vi "Write All.vi"(8 "Error In":errorcluster, 10 "Data":u8[](array[numeric]), 11 "SFTP File In":refnum<class "SFTP File.lvclass">) -> (0 "Error Out":errorcluster, 2 "Block Write Count":i64, 3 "SFTP File Out":refnum<class "SFTP File.lvclass">)   [LabVIEW 2018, in "Toolkit.lvlib" / "SFTP File.lvclass"]
doc: "Writes all of the bytes to a remote SFTP file in a series of smaller 30KB chunks, or blocks."
uses:
  SFTP File.lvclass
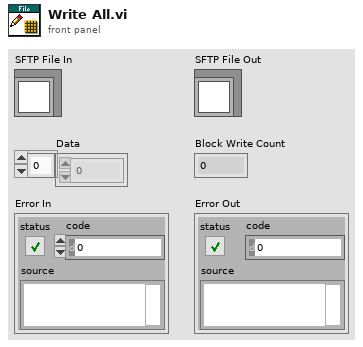
[diagram p1: front panel]
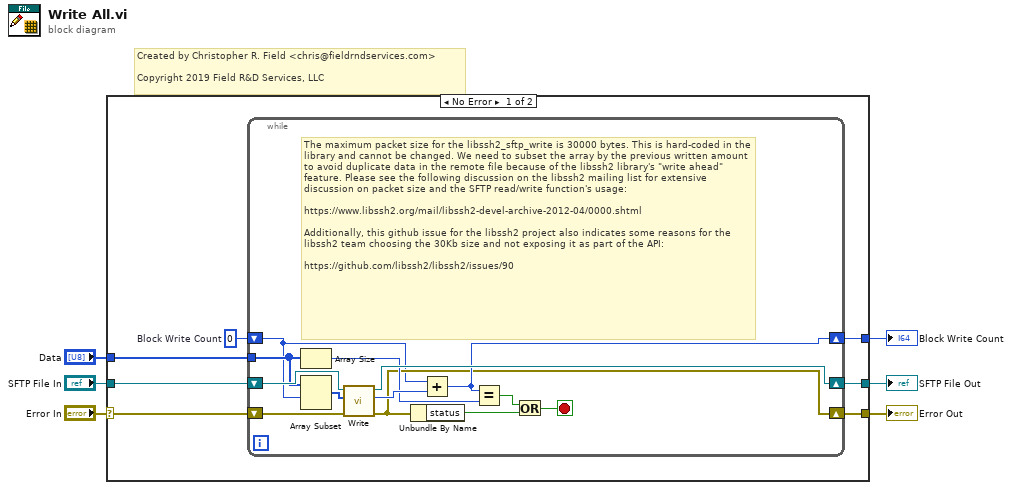
[diagram p0: block diagram]
diagram:
  # "Created by Christopher R. Field <chris@fieldrndservices.com>\n\nCopyright 2019 Field R&D Services, LLC"
  n1 = case shown="No Error" "Error In" {
    selector: "Error In" -> [w7 w27]
    tunnel: "Data" -> [w12 _]
    tunnel: "SFTP File In" -> [w11 w28]
    tunnel: [w10 _] -> w4
    tunnel: [w9 w28] -> w3
    tunnel: [w8 w27] -> w2
    frame No Error {
      w13 = i64 0  # Block Write Count
      n2 = while {
        tunnel: w12 -> [w20]
        shift-right: [w24] -> w9
        shift-left: w11 -> [w26]
        shift-right: [w16] -> w8
        shift-left: w7 -> [w25]
        shift-right: [w22] -> w10
        shift-left: w13 -> [w14]
        stop <- w17 stop-if-true
        # "The maximum packet size for the libssh2_sftp_write is 30000 bytes. This is hard-coded in the library and cannot be changed. We need to subset the array by the previous written amount to avoid duplicate data in the remote file because of the libssh2 library's \"write ahead\" feature. Please see the following discussion on the libssh2 mailing list for extensive discussion on packet size and the SFTP read/write function's usage:\n\nhttps://www.libssh2.org/mail/libssh2-devel-archive-2012-04/0000.shtml\n\nAdditionally, this github issue for the libssh2 project also indicates some reasons for the libssh2 team choosing the 30Kb size and not exposing it as part of the API:\n\nhttps://github.com/libssh2/libssh2/issues/90"
        n3 = Array Size(array=w20) -> (size(s)=w21:i32)
        n4 = Array Subset(array=w20, index=w14) -> (w19:u8[])  [unwired: 1 in]
        n5 = call "Write.vi"("Error In"=w25, "Data"=w19, "SFTP File In"=w26) -> ("Error Out"=w16:errorcluster, "Count"=w23:i64, "SFTP File Out"=w24:refnum<class "SFTP File.lvclass">)  [unwired: 6 in]
        n6 = Unbundle By Name(w16) -> ("status"=w15:bool)
        n7 = Add(x=w14, y=w23) -> (x+y=w22:i64)
        n8 = Equal?(x=w22, y=w21) -> (x = y?=w18:bool)
        n9 = Or(x=w18, y=w15) -> (x .or. y?=w17:bool)
      }
    }
    frame Error {
    }
  }
  "Block Write Count" <- w4
  "SFTP File Out" <- w3
  "Error Out" <- w2
